vi "Moment about Mean PtByPt.vi"(2 "initialize":bool, 3 "sample length":i32=100, 4 "order":i32=2, 5 "x":dbl format="%0.2f") -> (0 "error":i32, 1 "moment":dbl format="%0.2f")   [LabVIEW 2017, in "NI_PtbyPt.lvlib"]
doc: "Computes the <B>moment</B> about the mean using the specified <B>order</B>, m, for the set of input data points specified by <B>sample length</B>."
uses:
  <vilib>/ptbypt/NI_PtbyPt.lvlib
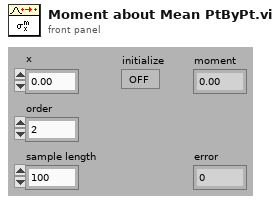
[diagram p1: front panel]
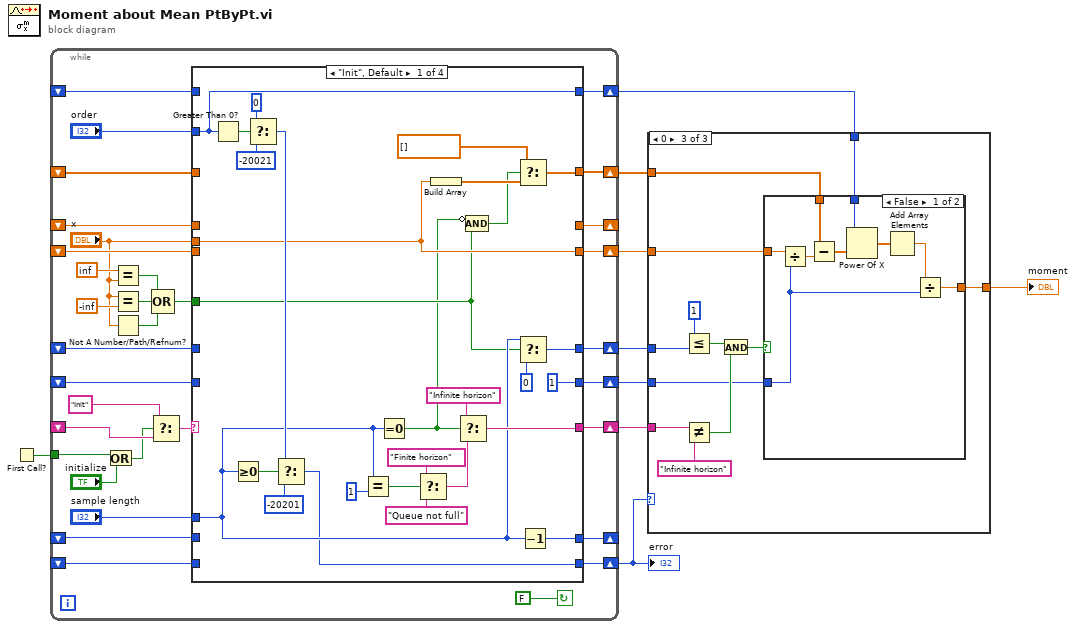
[diagram p0: block diagram]
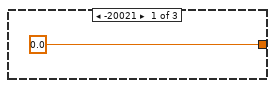
[diagram p2: hidden frame]
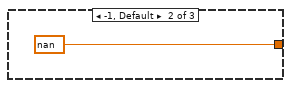
[diagram p3: hidden frame]
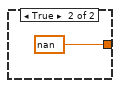
[diagram p4: hidden frame]
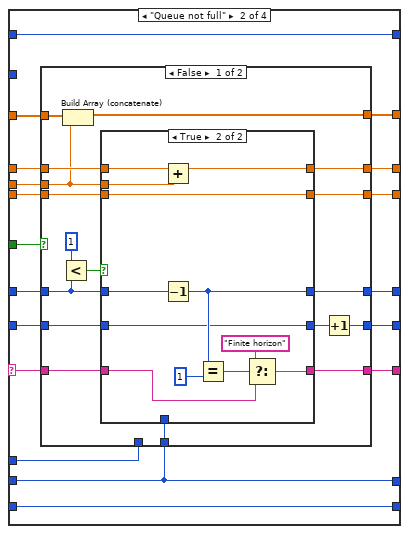
[diagram p5: hidden frame]
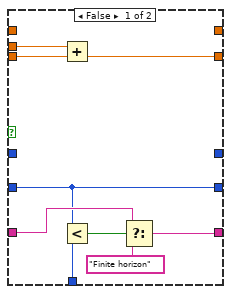
[diagram p6: hidden frame]
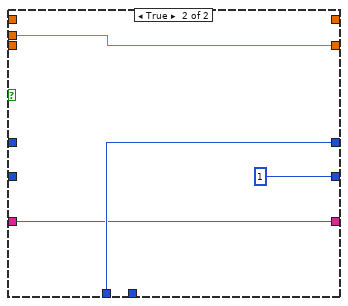
[diagram p7: hidden frame]
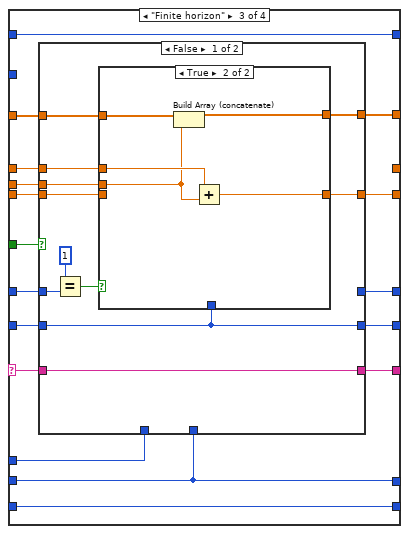
[diagram p8: hidden frame]
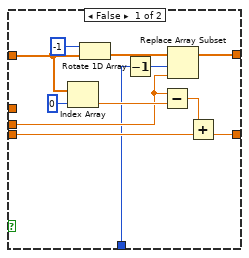
[diagram p9: hidden frame]
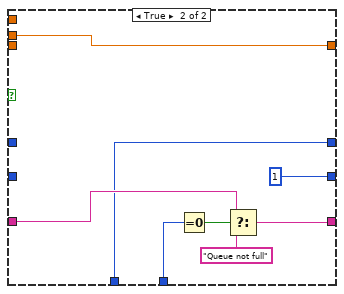
[diagram p10: hidden frame]
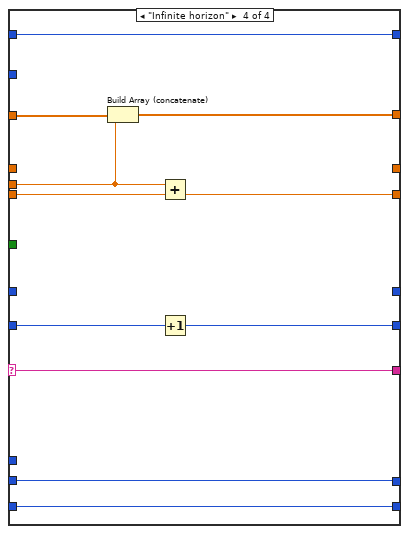
[diagram p11: hidden frame]
diagram:
  n1 = First Call?() -> (First Call?: T/F=w7:bool)
  n2 = while {
    shift-left: _ -> [w10]
    shift-right: [w24] -> w4
    tunnel: w7 -> [w28]
    shift-left: _ -> [w30]
    shift-right: [w31] -> _
    shift-left: _ -> [w34]
    shift-right: [w33] -> w3
    shift-left: _ -> [w36]
    shift-right: [w37] -> w9
    shift-left: _ -> [w38]
    shift-right: [w39] -> w2
    shift-left: _ -> [w42]
    shift-right: [w35] -> w5
    shift-right: [w17] -> w6
    shift-left: _ -> [w16]
    shift-right: [w15] -> _
    shift-left: _ -> [w14]
    shift-right: [w13] -> w1
    shift-left: _ -> [w12]
    stop <- FALSE continue-if-true
    n3 = Or(x=w28, y="initialize") -> (x .or. y?=w26:bool)
    n4 = Equal?(x=inf, y="x") -> (x = y?=w22:bool)
    n5 = Equal?(x="x", y=-inf) -> (x = y?=w21:bool)
    n6 = Not A Number/Path/Refnum?(number/path/refnum="x") -> (NaN/Path/Refnum?=w23:bool)
    n7 = Select(t="Init", s=w26, f=w42) -> (s? t:f=w40:string)
    n8 = Compound Arithmetic op=OR(w22, w21, w23) -> (w18:bool)
    n9 = case shown="\"Init\", Default" w40 {
      selector: w40 -> [_ w81 w140 w189]
      tunnel: [w47 w83 w142 w190] -> w39
      tunnel: w38 -> [_ w84 w141 w191]
      tunnel: "x" -> [w47 w85 w146 w183]
      tunnel: [1 w78 w135 w192] -> w37
      tunnel: w36 -> [_ w82 w145 w193]
      tunnel: [w57 w80 w139 w189] -> w35
      tunnel: w34 -> [_ w87 w143 w185]
      tunnel: [w51 w86 w144 w184] -> w33
      tunnel: "sample length" -> [w54 w72 w133 _]
      tunnel: [w63 w79 w134 w188] -> w31
      tunnel: w30 -> [_ w79 w134 w188]
      tunnel: "order" -> [w48 _ _ _]
      tunnel: [w48 w70 w130 w186] -> w24
      tunnel: w10 -> [_ w70 w130 w186]
      tunnel: w18 -> [w45 w77 w138 _]
      tunnel: [w53 w75 w132 _] -> w17
      tunnel: w16 -> [_ w76 w137 _]
      tunnel: [_ w74 _ _] -> w15
      tunnel: w14 -> [_ w73 w136 _]
      tunnel: [w49 w71 w131 w187] -> w13
      tunnel: w12 -> [_ w71 w131 w187]
      frame "Init", Default {
        n10 = Greater Than 0?(x=w48) -> (x > 0?=w62:bool)
        n11 = Greater Or Equal To 0?(x=w54) -> (x >= 0?=w64:bool)
        n12 = Select(t=0, s=w62, f=-20021) -> (s? t:f=w59:i32)
        n13 = Select(t=w59, s=w64, f=-20201) -> (s? t:f=w49:i32)
        n14 = Equal?(x=w54, y=1) -> (x = y?=w67:bool)
        n15 = Equal To 0?(x=w54) -> (x = 0?=w44:bool)
        n16 = Select(t="Finite horizon", s=w67, f="Queue not full") -> (s? t:f=w56:string)
        n17 = Build Array(w47) -> (w46:dbl[])
        n18 = Select(t="Infinite horizon", s=w44, f=w56) -> (s? t:f=w57:string)
        n19 = Compound Arithmetic op=AND(invert w44, w45) -> (w43:bool)
        n20 = Select(t=dbl[] [] ("f"), s=w43, f=w46) -> (s? t:f=w51:dbl[])
        n21 = Select(t=w54, s=w45, f=0) -> (s? t:f=w53:i32)
        n22 = Decrement(x=w54) -> (x-1=w63:i32)
      }
      frame "Queue not full" {
        n23 = case shown="False" w77 {
          tunnel: w87 -> [w104 _]
          tunnel: [w103 _] -> w86
          tunnel: w85 -> [w90 w126]
          tunnel: w84 -> [w102 _]
          tunnel: [w101 w126] -> w83
          tunnel: w82 -> [w100 _]
          tunnel: w81 -> [w99 w127]
          tunnel: [w98 w127] -> w80
          tunnel: w79 -> [w97 _]
          tunnel: [w88 1] -> w78
          tunnel: w76 -> [w94 _]
          tunnel: [w93 w129] -> w75
          tunnel: [w92 _] -> w74
          tunnel: w73 -> [w91 _]
          tunnel: w72 -> [_ w129]
          frame False {
            n24 = Less?(x=1, y=w94) -> (x < y?=w95:bool)
            n25 = Build Array (concatenate)(w104, w90) -> (w103:dbl[])
            n26 = case shown="True" w95 {
              tunnel: w90 -> [w107 w115]
              tunnel: w102 -> [w113 w118]
              tunnel: [w106 w118] -> w101
              tunnel: w100 -> [w105 w114]
              tunnel: w99 -> [w111 w119]
              tunnel: [w109 w120] -> w98
              tunnel: w97 -> [w108 _]
              tunnel: [w105 w114] -> w89
              tunnel: w94 -> [_ w122]
              tunnel: [_ w121] -> w93
              tunnel: [_ w116] -> w92
              tunnel: w91 -> [_ w117]
              frame False {
                n27 = Add(x=w107, y=w113) -> (x+y=w106:dbl)
                n28 = Less?(x=w105, y=w108) -> (x < y?=w112:bool)
                n29 = Select(t=w111, s=w112, f="Finite horizon") -> (s? t:f=w109:string)
              }
              frame True {
                n30 = Add(x=w117, y=w115) -> (x+y=w116:dbl)
                n31 = Decrement(x=w122) -> (x-1=w121:i32)
                n32 = Equal?(x=w121, y=1) -> (x = y?=w125:bool)
                n33 = Select(t="Finite horizon" ("f"), s=w125, f=w119) -> (s? t:f=w120:string)
              }
            }
            n34 = Increment(x=w89) -> (x+1=w88:i32)
          }
          frame True {
          }
        }
      }
      frame "Finite horizon" {
        n35 = case shown="False" w138 {
          tunnel: w146 -> [w147 w175]
          tunnel: w145 -> [w148 _]
          tunnel: [w157 _] -> w144
          tunnel: w143 -> [w156 _]
          tunnel: [w155 w175] -> w142
          tunnel: w141 -> [w154 _]
          tunnel: w140 -> [w153 w177]
          tunnel: [w153 w179] -> w139
          tunnel: w137 -> [w151 _]
          tunnel: w136 -> [w149 _]
          tunnel: [w148 1] -> w135
          tunnel: w134 -> [_ w178]
          tunnel: w133 -> [_ w176]
          tunnel: [_ w176] -> w132
          frame False {
            n36 = Equal?(x=1, y=w151) -> (x = y?=w150:bool)
            n37 = case shown="True" w150 {
              tunnel: w147 -> [w160 w170]
              tunnel: w148 -> [w158 _]
              tunnel: [w165 w173] -> w157
              tunnel: w156 -> [w163 w174]
              tunnel: [w159 w171] -> w155
              tunnel: w154 -> [w161 _]
              tunnel: w149 -> [_ w172]
              frame False {
                n38 = Index Array(array=w163, index=0 ("Index")) -> (element=w164:dbl)
                n39 = Rotate 1D Array(1:w163, 2:i16 -1 ("n")) -> (0:w167:dbl[])
                n40 = Decrement(x=w158) -> (x-1=w166:i32)
                n41 = Subtract(x=w160, y=w164) -> (x-y=w162:dbl)
                n42 = Replace Array Subset(array=w167, new element=w160, index=w166) -> (w165:dbl[])
                n43 = Add(x=w162, y=w161) -> (x+y=w159:dbl)
              }
              frame True {
                n44 = Build Array (concatenate)(w174, w170) -> (w173:dbl[])
                n45 = Add(x=w172, y=w170) -> (x+y=w171:dbl)
              }
            }
          }
          frame True {
            n46 = Equal To 0?(x=w178) -> (x = 0?=w182:bool)
            n47 = Select(t=w177, s=w182, f="Queue not full") -> (s? t:f=w179:string)
          }
        }
      }
      frame "Infinite horizon" {
        n48 = Build Array (concatenate)(w185, w183) -> (w184:dbl[])
        n49 = Add(x=w183, y=w191) -> (x+y=w190:dbl)
        n50 = Increment(x=w193) -> (x+1=w192:i32)
      }
    }
  }
  "error" <- w1
  n51 = case shown="0" w1 {
    tunnel: w9 -> [_ _ w198]
    tunnel: [0.0 nan w197] -> w8
    tunnel: w6 -> [_ _ w207]
    tunnel: w5 -> [_ _ w205]
    tunnel: w4 -> [_ _ w201]
    tunnel: w3 -> [_ _ w199]
    tunnel: w2 -> [_ _ w200]
    frame -20021 {
    }
    frame -1, Default {
    }
    frame 0 {
      n52 = Less Or Equal?(x=1, y=w207) -> (x <= y?=w203:bool)
      n53 = Not Equal?(x=w205, y="Infinite horizon") -> (x != y?=w202:bool)
      n54 = And(x=w203, y=w202) -> (x .and. y?=w196:bool)
      n55 = case shown="False" w196 {
        tunnel: w201 -> [w216 _]
        tunnel: w200 -> [w215 _]
        tunnel: w199 -> [w214 _]
        tunnel: w198 -> [w209 _]
        tunnel: [w208 nan] -> w197
        frame False {
          n56 = Divide(x=w215, y=w209) -> (x/y=w213:dbl)
          n57 = Subtract(x=w214, y=w213) -> (x-y=w212:dbl[])
          n58 = Power Of X(1:w212, 2:w216) -> (0:w211:dbl[])
          n59 = Add Array Elements(numeric array=w211) -> (sum=w210:dbl)
          n60 = Divide(x=w210, y=w209) -> (x/y=w208:dbl)
        }
        frame True {
        }
      }
    }
  }
  "moment" <- w8
